vi "rotate-body.vi"(8 "Error In":errorcluster caption="错误输入", 10 "Angle":i32, 11 "SceneObject输入":refnum<vi>) -> (0 "Error Out":errorcluster caption="错误输出", 3 "Object Out":refnum<vi> caption="场景对象")   [LabVIEW 2013]
uses:
  <vilib>/picture/3D Picture Control/NI_3D Picture Control.lvlib
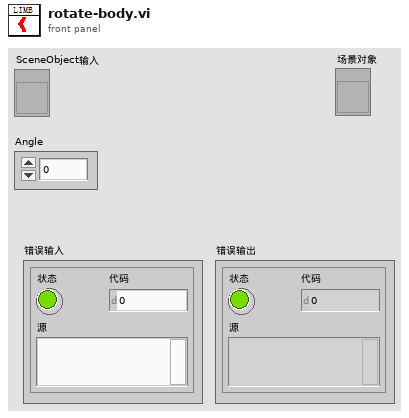
[diagram p1: front panel]
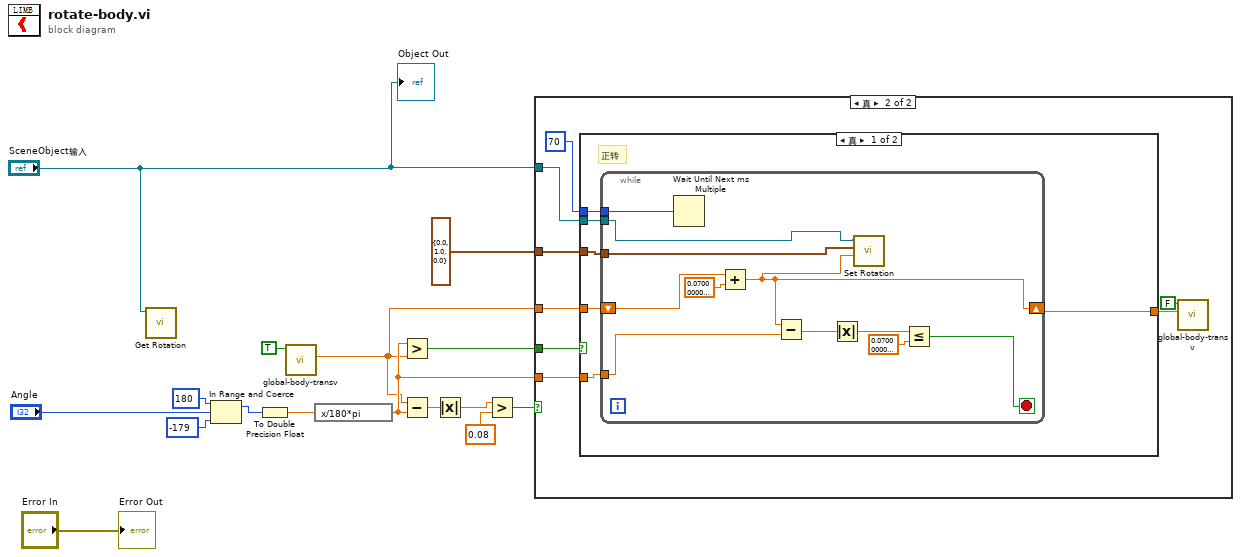
[diagram p0: block diagram]
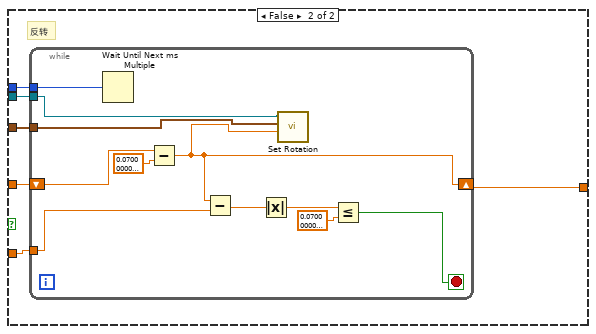
[diagram p3: hidden frame]
diagram:
  n1 = call <vilib>:"Get Rotation.vi"("Scene Object"="SceneObject输入") -> ()  [unwired: 7 in, 4 out]
  n2 = In Range and Coerce(upper limit=180 ("上限"), x="Angle", lower limit=-179 ("下限")) -> (coerced(x)=w12:i32)  [unwired: 1 out]
  n3 = To Double Precision Float(number=w12) -> (double precision float=w15:dbl)
  n4 = call "global-body-transv.vi"("Read?"=TRUE) -> ("rad out"=w2:dbl)  [unwired: 9 in, 1 out]
  n5 = expression code="x/180*pi"(w15) -> (w3:dbl)
  n6 = Greater?(x=w3, y=w2) -> (0:w4:bool)
  n7 = Subtract(x=w2, y=w3) -> (x-y=w16:dbl)
  n8 = Absolute Value(x=w16) -> (abs(x)=w7:dbl)
  n9 = Greater?(x=w7, y=0.08) -> (0:w6:bool)
  n10 = case shown="真" w6 {
    tunnel: "SceneObject输入" -> [_ w24]
    tunnel: w4 -> [_ w23]
    tunnel: w2 -> [_ w22]
    tunnel: w3 -> [_ w20]
    tunnel: cluster{"X":sgl, "Y":sgl, "Z":sgl} {"X"=0.0, "Y"=1.0, "Z"=0.0} ("Axis") -> [_ w17]
    frame False {
    }
    frame True {
      n11 = case shown="真" w23 {
        tunnel: w24 -> [w30 w47]
        tunnel: w22 -> [w29 w46]
        tunnel: u32 70 ("毫秒倍数") -> [w28 w45]
        tunnel: w20 -> [w27 w44]
        tunnel: [w26 w43] -> w18
        tunnel: w17 -> [w25 w42]
        frame True {
          # "正转"
          n12 = while {
            tunnel: w30 -> [w33]
            shift-right: [w32] -> w26
            shift-left: w29 -> [w39]
            tunnel: w28 -> [w41]
            tunnel: w27 -> [w38]
            tunnel: w25 -> [w31]
            stop <- w34 stop-if-true
            n13 = Wait Until Next ms Multiple(millisecond multiple=w41) -> ()  [unwired: 1 out]
            n14 = Add(x=w39, y=sgl 0.07) -> (x+y=w32:dbl)
            n15 = Subtract(x=w32, y=w38) -> (x-y=w35:dbl)
            n16 = Absolute Value(x=w35) -> (abs(x)=w37:dbl)
            n17 = call <vilib>:"Set Rotation.vi"("Angle"=w32, "Axis"=w31, "Scene Object"=w33) -> ()  [unwired: 7 in, 2 out]
            n18 = Less Or Equal?(x=w37, y=sgl 0.07) -> (x <= y?=w34:bool)
          }
        }
        frame False {
          # "反转"
          n19 = while {
            tunnel: w47 -> [w49]
            shift-right: [w50] -> w43
            shift-left: w46 -> [w56]
            tunnel: w45 -> [w58]
            tunnel: w44 -> [w55]
            tunnel: w42 -> [w48]
            stop <- w51 stop-if-true
            n20 = Wait Until Next ms Multiple(millisecond multiple=w58) -> ()  [unwired: 1 out]
            n21 = Subtract(x=w56, y=sgl 0.07) -> (x-y=w50:dbl)
            n22 = Subtract(x=w50, y=w55) -> (x-y=w52:dbl)
            n23 = Absolute Value(x=w52) -> (abs(x)=w54:dbl)
            n24 = call <vilib>:"Set Rotation.vi"("Angle"=w50, "Axis"=w48, "Scene Object"=w49) -> ()  [unwired: 7 in, 2 out]
            n25 = Less Or Equal?(x=w54, y=sgl 0.07) -> (x <= y?=w51:bool)
          }
        }
      }
      n26 = call "global-body-transv.vi"("rad"=w18, "Read?"=FALSE) -> ()  [unwired: 8 in, 2 out]
    }
  }
  "Error Out" <- "Error In"
  "Object Out" <- "SceneObject输入"
